vi "Get Info.vi"(6 "Variant in":variant, 7 "Shift Pressed?":bool, 8 "error in (no error)":errorcluster, 10 "QD Combo Box Ref":refnum<vi>, 11 "QD Launch VI Ref":refnum<vi>) -> (0 "error out":errorcluster, 4 "Variant out":variant)   [LabVIEW 2019]
doc: "Gets information depending on the selection:\n\nCreated by: Ryan Pacini\n\nDefault Shortcut - [G]"
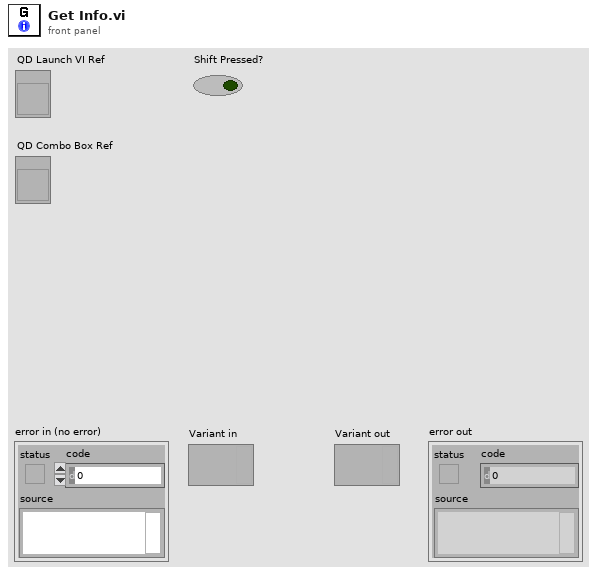
[diagram p1: front panel]
types:
  T1 = typedef "LVBoundsTypeDef.ctl" = cluster{"Width":u32, "Height":u32}
  T2 = typedef "LVRectTypeDef.ctl" = cluster{"Left":i16, "Top":i16, "Right":i16, "Bottom":i16}
  T3 = typedef "LVPositionTypeDef.ctl" = cluster{"Left":i32, "Top":i32}
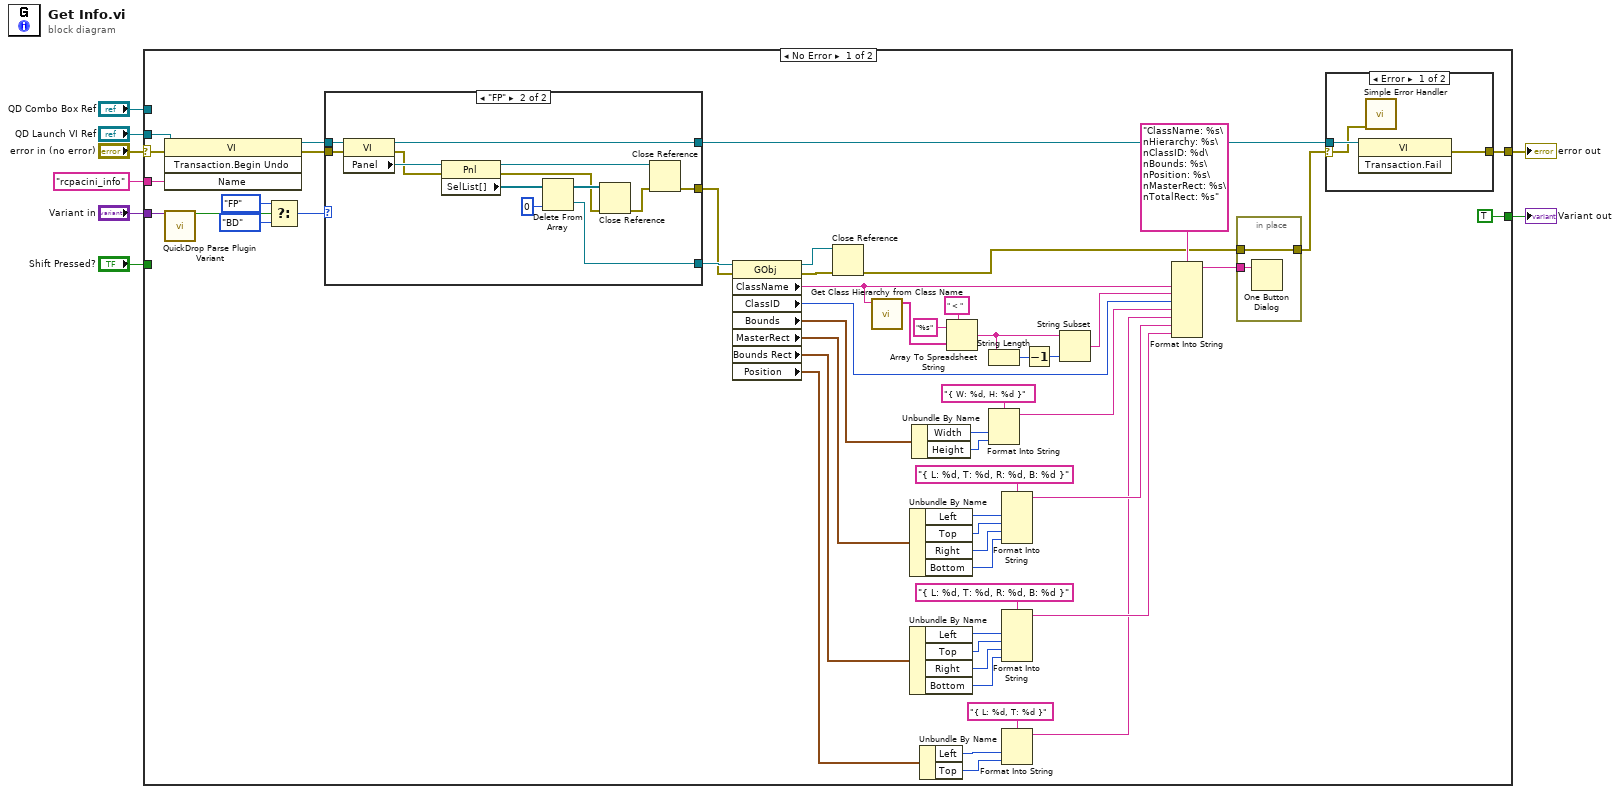
[diagram p0: block diagram]
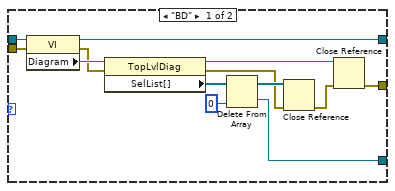
[diagram p2: hidden frame]
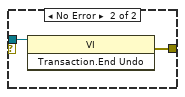
[diagram p3: hidden frame]
diagram:
  n1 = case shown="No Error" "error in (no error)" {
    selector: "error in (no error)" -> [w62 w96]
    tunnel: [w61 w96] -> w3
    tunnel: "QD Launch VI Ref" -> [w57 _]
    tunnel: "rcpacini_info" ("Undo Name") -> [w60 _]
    tunnel: "Variant in" -> [w58 _]
    tunnel: [TRUE _] -> w4
    tunnel: "QD Combo Box Ref" -> [_ _]
    tunnel: "Shift Pressed?" -> [_ _]
    frame No Error {
      n2 = invoke class="VI" method="Transaction.Begin Undo"(reference=w57, error in=w62, "Name"=w60) -> (reference out=w56:refnum<vi>, error out=w55:errorcluster)  [unwired: 1 in, 2 out]
      n3 = call <vilib>:"QuickDrop Parse Plugin Variant.vi"("QDKS Variant in"=w58) -> ("QD Launch VI Panel?"=w52:bool)  [unwired: 12 in, 2 out]
      n4 = Select(t=enum8{"FP", "BD"}."FP" ("Panel"), s=w52, f=enum8{"FP", "BD"}."BD" ("Panel")) -> (s? t:f=w24:enum8{"FP", "BD"})
      n5 = case shown="\"FP\"" w24 {
        tunnel: w56 -> [w77 w90]
        tunnel: w55 -> [w76 w89]
        tunnel: [w71 w84] -> w30
        tunnel: [w66 w79] -> w29
        tunnel: [w65 w78] -> w27
        frame "BD" {
          n6 = property class="VI"(reference=w77, error in=w76) -> (reference out=w66:refnum<vi>, error out=w74:errorcluster, "Diagram"=w75:refnum<vi>)
          n7 = property class="TopLvlDiag"(reference=w75, error in=w74) -> (reference out=w68:refnum<vi>, error out=w69:errorcluster, "SelList[]"=w73:refnum<vi>[])
          n8 = Delete From Array(array=w73, index=0) -> (deleted portion=w71:refnum<vi>, array with subset deleted=w70:refnum<vi>[])  [unwired: 1 in]
          n9 = Close Reference(reference=w70, error in (no error)=w69) -> (error out=w67:errorcluster)
          n10 = Close Reference(reference=w68, error in (no error)=w67) -> (error out=w65:errorcluster)
        }
        frame "FP" {
          n11 = property class="VI"(reference=w90, error in=w89) -> (reference out=w79:refnum<vi>, error out=w87:errorcluster, "Panel"=w88:refnum<vi>)
          n12 = property class="Pnl"(reference=w88, error in=w87) -> (reference out=w81:refnum<vi>, error out=w82:errorcluster, "SelList[]"=w86:refnum<vi>[])
          n13 = Delete From Array(array=w86, index=0) -> (deleted portion=w84:refnum<vi>, array with subset deleted=w83:refnum<vi>[])  [unwired: 1 in]
          n14 = Close Reference(reference=w83, error in (no error)=w82) -> (error out=w80:errorcluster)
          n15 = Close Reference(reference=w81, error in (no error)=w80) -> (error out=w78:errorcluster)
        }
      }
      n16 = property class="GObj"(reference=w30, error in=w27) -> (reference out=w19:refnum<vi>, error out=w28:errorcluster, "ClassName"=w10:string, "ClassID"=w11:u32, "Bounds"=w51:T1, "MasterRect"=w43:T2, "Bounds Rect"=w33:T2, "Position"=w20:T3)
      n17 = Close Reference(reference=w19, error in (no error)=w28) -> (error out=w26:errorcluster)
      n18 = call <vilib>:"Get Class Hierarchy from Class Name.vi"("Class Name"=w10) -> ("Class Hierarchy"=w18:string[])  [unwired: 9 in, 1 out]
      n19 = Unbundle By Name(w43) -> ("Left"=w44:i16, "Top"=w45:i16, "Right"=w41:i16, "Bottom"=w40:i16)
      n20 = Unbundle By Name(w33) -> ("Left"=w35:i16, "Top"=w34:i16, "Right"=w37:i16, "Bottom"=w38:i16)
      n21 = Unbundle By Name(w51) -> ("Width"=w50:u32, "Height"=w49:u32)
      n22 = Unbundle By Name(w20) -> ("Left"=w22:i32, "Top"=w23:i32)
      n23 = Array To Spreadsheet String(delimiter (Tab)=" < ", array=w18, 3:"%s" ("format string")) -> (spreadsheet string=w15:string)
      n24 = String Length(string=w15) -> (length=w14:i32)
      n25 = Format Into String(format string="{ W: %d, H: %d }", w50, w49) -> (resulting string=w47:string)  [unwired: 2 in, 1 out]
      n26 = Format Into String(format string="{ L: %d, T: %d, R: %d, B: %d }", w44, w45, w41, w40) -> (resulting string=w39:string)  [unwired: 2 in, 1 out]
      n27 = Format Into String(format string="{ L: %d, T: %d, R: %d, B: %d }", w35, w34, w37, w38) -> (resulting string=w32:string)  [unwired: 2 in, 1 out]
      n28 = Format Into String(format string="{ L: %d, T: %d }", w22, w23) -> (resulting string=w9:string)  [unwired: 2 in, 1 out]
      n29 = Decrement(x=w14) -> (x-1=w13:i32)
      n30 = String Subset(string=w15, length (rest)=w13) -> (substring=w12:string)  [unwired: 1 in]
      n31 = Format Into String(format string="ClassName: %s\nHierarchy: %s\nClassID: %d\nBounds: %s\nPosition: %s\nMasterRect: %s\nTotalRect: %s", w10, w12, w11, w47, w9, w39, w32) -> (resulting string=w31:string)  [unwired: 2 in, 1 out]
      n32 = in-place {
        in-place-border: w31 -> [w64]
        in-place-border: [w63] -> w25
        in-place-border: w26 -> [w63]
        n33 = One Button Dialog(message=w64) -> ()  [unwired: 1 in, 1 out]
      }
      n34 = case shown="Error" w25 {
        selector: w25 -> [w91 _]
        tunnel: w29 -> [w92 w94]
        tunnel: [w93 w95] -> w61
        frame Error {
          n35 = invoke class="VI" method="Transaction.Fail"(reference=w92) -> (error out=w93:errorcluster)  [unwired: 2 in, 2 out]
          n36 = call <vilib>:"Simple Error Handler.vi"("error in (no error)"=w91) -> ()  [unwired: 4 in, 5 out]
        }
        frame No Error {
          n37 = invoke class="VI" method="Transaction.End Undo"(reference=w94) -> (error out=w95:errorcluster)  [unwired: 2 in, 2 out]
        }
      }
    }
    frame Error {
    }
  }
  "error out" <- w3
  "Variant out" <- w4
